vi "unregisterAll.vi"(8 "error in (no error)":errorcluster, 11 "SAL_Listener in":refnum<class "SAL_Listener.lvclass">) -> (0 "error out":errorcluster, 3 "SAL_Listener out":refnum<class "SAL_Listener.lvclass">)   [LabVIEW 2016, in "SAL_Listener.lvclass"]
uses:
  SAL_Listener.lvclass
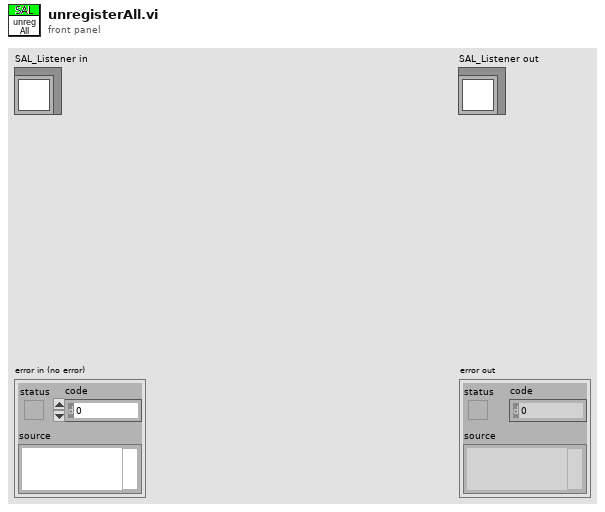
[diagram p1: front panel]
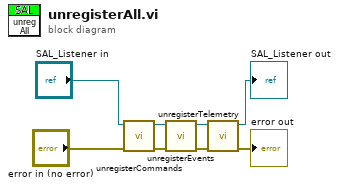
[diagram p0: block diagram]
diagram:
  n1 = call "unregisterCommands.vi"("error in (no error)"="error in (no error)", "SAL_Listener in"="SAL_Listener in") -> ("error out"=w2:errorcluster, "SAL_Listener out"=w4:refnum<class "SAL_Listener.lvclass">)  [unwired: 8 in]
  n2 = call "unregisterEvents.vi"("error in (no error)"=w2, "SAL_Listener in"=w4) -> ("error out"=w1:errorcluster, "SAL_Listener out"=w3:refnum<class "SAL_Listener.lvclass">)  [unwired: 8 in]
  n3 = call "unregisterTelemetry.vi"("error in (no error)"=w1, "SAL_Listener in"=w3) -> ("error out"=→"error out":errorcluster, "SAL_Listener out"=→"SAL_Listener out":refnum<class "SAL_Listener.lvclass">)  [unwired: 8 in]
